vi "Set Bitrate.vi"(8 "error in (no error)":errorcluster, 10 "Bitrates":T1, 11 "uCAN in":refnum<class "uCAN.lvclass">) -> (0 "error out":errorcluster, 3 "uCAN out":refnum<class "uCAN.lvclass">)   [LabVIEW 2021, in "uCanDriver.lvlib" / "uCAN.lvclass"]
uses:
  uCAN.lvclass
  typedefs/bitrates.ctl
  uCAN.lvclass/uCAN.ctl
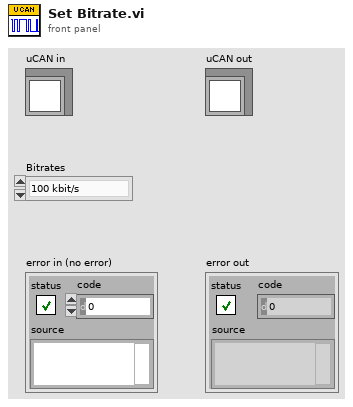
[diagram p1: front panel]
types:
  T1 = typedef "uCanDriver.lvlib/uCAN.lvclass/bitrates.ctl" = enum16{"100 kbit/s", "125 kbit/s", "250 kbit/s", "500 kbit/s", "800 kbit/s", "1 Mbit/s"}
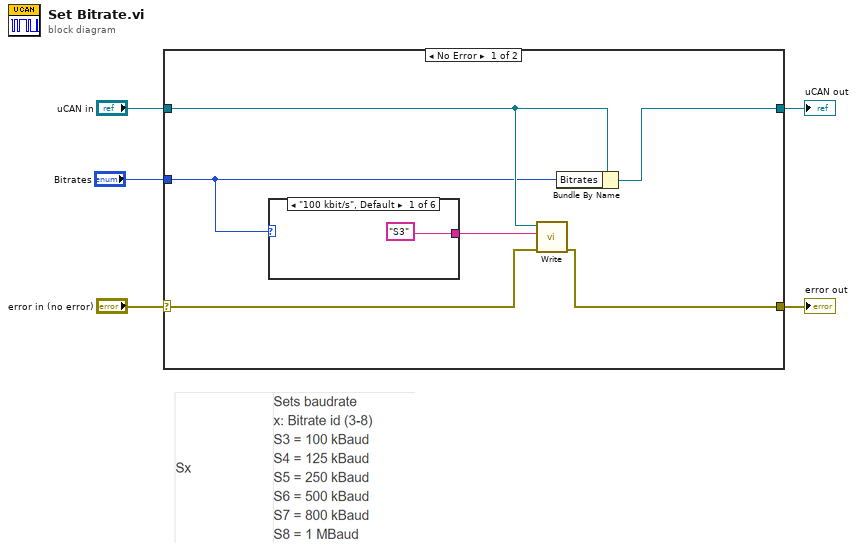
[diagram p0: block diagram]
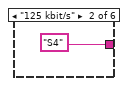
[diagram p2: hidden frame]
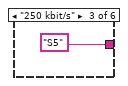
[diagram p3: hidden frame]
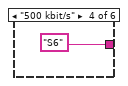
[diagram p4: hidden frame]
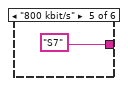
[diagram p5: hidden frame]
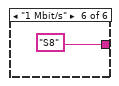
[diagram p6: hidden frame]
diagram:
  n1 = case shown="No Error" "error in (no error)" {
    selector: "error in (no error)" -> [w7 w19]
    tunnel: [w6 w19] -> w4
    tunnel: [w11 w18] -> w2
    tunnel: "uCAN in" -> [w10 w18]
    tunnel: "Bitrates" -> [w9 _]
    frame No Error {
      n2 = case shown="\"100 kbit/s\", Default" w9 {
        tunnel: ["S3" "S4" "S5" "S6" "S7" "S8"] -> w8
        frame "100 kbit/s", Default {
        }
        frame "125 kbit/s" {
        }
        frame "250 kbit/s" {
        }
        frame "500 kbit/s" {
        }
        frame "800 kbit/s" {
        }
        frame "1 Mbit/s" {
        }
      }
      n3 = call "Write.vi"("error in (no error)"=w7, "write buffer"=w8, "uCAN in"=w10) -> ("error out"=w6:errorcluster)  [unwired: 8 in]
      n4 = Bundle By Name(cluster=w10, "Bitrates"=w9) -> (w11:refnum<class "uCAN.lvclass">)
    }
    frame Error {
    }
  }
  "error out" <- w4
  "uCAN out" <- w2
